vi "TimeoutDialog.vi"(1 "message 2":string="Hello This is the message") -> ()   [LabVIEW 2020]
panel:
  in  "OK Button":bool
  out "message":string="Hello This is the message"
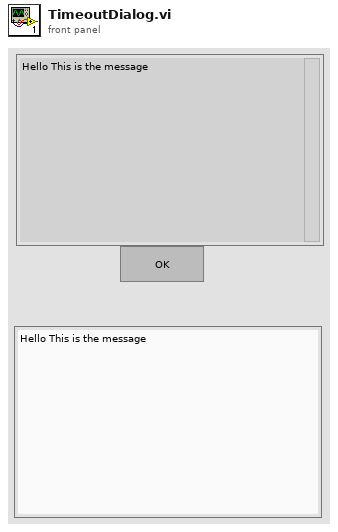
[diagram p1: front panel]
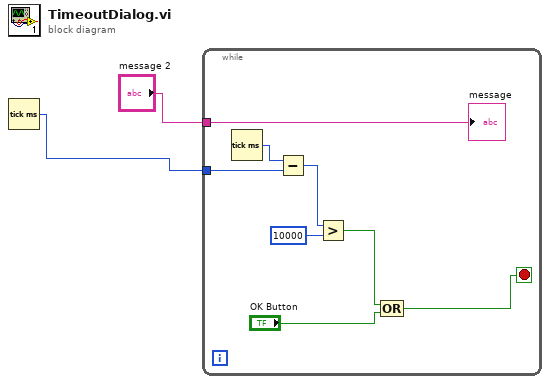
[diagram p0: block diagram]
diagram:
  n1 = Tick Count (ms)() -> (millisecond timer value=w2:u32)
  n2 = while {
    tunnel: w2 -> [w10]
    tunnel: "message 2" -> [w3]
    stop <- w4 stop-if-true
    n3 = Tick Count (ms)() -> (millisecond timer value=w7:u32)
    n4 = Subtract(x=w7, y=w10) -> (x-y=w9:u32)
    n5 = Greater?(x=w9, y=u32 10000) -> (0:w6:bool)
    n6 = Compound Arithmetic op=OR(w6, "OK Button") -> (w4:bool)
    "message" <- w3
  }
